vi "Configuration Write Do.vi"(7 "Digit Resolution(5½)":T1=enum."5½", 8 "error in (no error)":errorcluster, 9 "Range":dbl, 10 "Function":T2, 11 "NI DMM Driver in":refnum<class "DMM.NI.lvclass">) -> (0 "error out":errorcluster, 1 "Success?":bool, 3 "NI DMM Driver out":refnum<class "DMM.NI.lvclass">)   [LabVIEW 2020, in "NI DMM Driver.lvlib" / "DMM.NI.lvclass"]
doc: "Configure the DMM Function, Range and Resolution."
uses:
  DMM.NI.lvclass
  PPL/HDH.Driver.DMM.lvlibp/Controls/Ctl_Function.ctl
  PPL/HDH.Driver.DMM.lvlibp/Controls/Ctl_DigitResolution.ctl
  DMM.NI.lvclass/DMM.NI.ctl
  <instrlib>/niDMM/nidmm.llb/niDMM Configure Measurement Digits.vi
  PPL/HDH.Driver.DMM.lvlibp
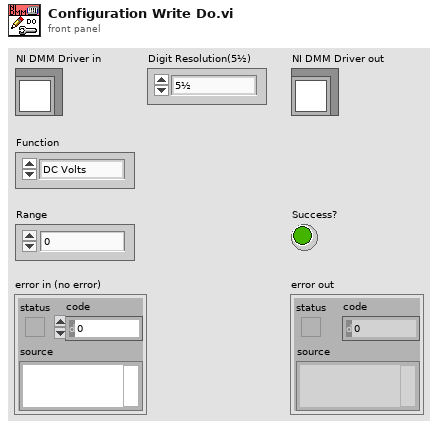
[diagram p1: front panel]
types:
  T1 = typedef "HDH.Driver.DMM.lvlibp/Ctl_DigitResolution.ctl" = enum8{"3½", "4½", "5½", "6½", "7½"}
  T2 = typedef "HDH.Driver.DMM.lvlibp/Ctl_Function.ctl" = enum8{"DC Volts", "AC Volts", "DC Current", "AC Current", "2-wire Resistance", "4-wire Resistance", "Diode", "Frequency", "Period", "AC Volts DC Coupled", "Capacitance", "Inductance", "Temperature"}
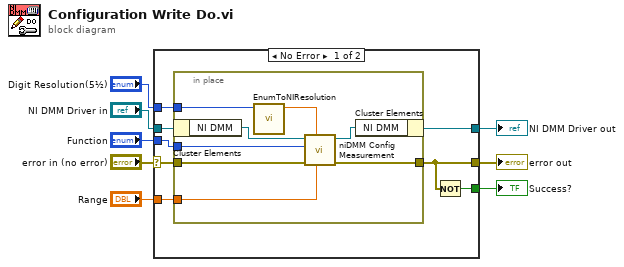
[diagram p0: block diagram]
diagram:
  n1 = case shown="No Error" "error in (no error)" {
    selector: "error in (no error)" -> [w14 w26]
    tunnel: [w13 w26] -> w4
    tunnel: [w15 w25] -> w7
    tunnel: "NI DMM Driver in" -> [w16 w25]
    tunnel: [w12 _] -> w6
    tunnel: "Function" -> [w11 _]
    tunnel: "Range" -> [w10 _]
    tunnel: "Digit Resolution(5½)" -> [w9 _]
    frame No Error {
      n2 = in-place {
        in-place-border: w14 -> [w22]
        in-place-border: [w21] -> w13
        in-place-border: w11 -> [w20]
        in-place-border: w10 -> [w19]
        in-place-border: w9 -> [w18]
        n3 = in-place-cluster #1(w16) -> ("NI DMM"=w24:refnum<k15>)
        n4 = call "EnumToNIResolution.vi"("Digit Resolution(5½)"=w18) -> ("NI Resolution"=w17:dbl)  [unwired: 10 in]
        n5 = call-poly <instrlib>:"niDMM Config Measurement.vi"("Range"=w19, "Resolution in Digits"=w17, "error in (no error)"=w22, "Function"=w20, "instrument handle"=w24) -> ("error out"=w21:errorcluster, "instrument handle out"=w23:refnum<k15>)  [unwired: 5 in]
        n6 = in-place-cluster #1("NI DMM"=w23) -> (w15:refnum<class "DMM.NI.lvclass">)
      }
      n7 = Not(x=w13) -> (.not. x?=w12:bool)
    }
    frame Error {
    }
  }
  "error out" <- w4
  "NI DMM Driver out" <- w7
  "Success?" <- w6
